vi "VIPM Increment Patch.vi"(8 "error in (no error)":errorcluster, 10 "selected path":path) -> (0 "error out":errorcluster, 2 "VI Package Build Spec Data":T1)   [LabVIEW 2019, in "Build.lvlib"]
uses:
  Build.lvlib
  <vilib>/JKI/VIPM API/command-line/support/VI Package Build Spec Data Cluster_vipm_api.ctl
  <vilib>/JKI/VIPM API/command-line/support/Version Info Cluster_vipm_api.ctl
  <vilib>/JKI/VIPM API/VIPM API_vipm_api.lvlib
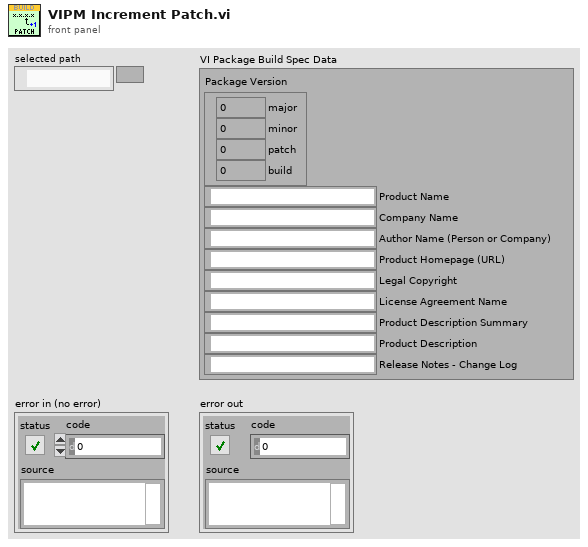
[diagram p1: front panel]
types:
  T1 = typedef "VIPM API_vipm_api.lvlib/VI Package Build Spec Data Cluster_vipm_api.ctl" = cluster{"Package Version":T2, "Product Name":string, "Company Name":string, "Author Name (Person or Company)":string, "Product Homepage (URL)":string, "Legal Copyright":string, "License Agreement Name":string, "Product Description Summary":string, "Product Description":string, "Release Notes - Change Log":string}
  T2 = typedef "VIPM API_vipm_api.lvlib/Version Info Cluster_vipm_api.ctl" = cluster{"major":u32, "minor":u32, "patch":u32, "build":u32}
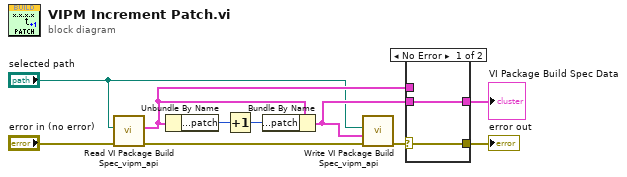
[diagram p0: block diagram]
diagram:
  n1 = call <vilib>:"Read VI Package Build Spec_vipm_api.vi"("error in (no error)"="error in (no error)", "Path to VIPB File"="selected path") -> ("error out"=w8:errorcluster, "VI Package Build Spec Data"=w3:T1)  [unwired: 8 in]
  n2 = Unbundle By Name(w3) -> ("Package Version.patch"=w10:u32)
  n3 = Increment(x=w10) -> (x+1=w9:u32)
  n4 = Bundle By Name(cluster=w3, "Package Version.patch"=w9) -> (w2:T1)
  n5 = call <vilib>:"Write VI Package Build Spec_vipm_api.vi"("error in (no error)"=w8, "VI Package Build Spec Data"=w2, "Path to VIPB File"="selected path") -> ("error out"=w5:errorcluster)  [unwired: 8 in]
  n6 = case shown="No Error" w5 {
    selector: w5 -> [w12 w14]
    tunnel: [w12 w14] -> w6
    tunnel: [w11 w13] -> w4
    tunnel: w2 -> [w11 _]
    tunnel: w3 -> [_ w13]
    frame No Error {
    }
    frame Error {
    }
  }
  "error out" <- w6
  "VI Package Build Spec Data" <- w4
